vi "Dejar Caja Global.vi"() -> ()   [LabVIEW 2014]
panel:
  in  "Sacar caja":bool
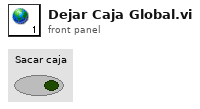
[diagram p1: front panel]
diagram:
